vi "Status TCU Module.vi"(8 "error in (no error)":errorcluster, 11 "?":T1={"State"=enum."Idle", "Start Time"=timestamp(0 s since 1904-01-01), "Configuration"={"Cycle Period"=0.0, "Setpoint Entry"=0.0, "Output Device"=enum."Default", "Huber Ministat 230 Settings"={"VISA resource name"="", "Simulated?"=FALSE}, "Lauda Settings"={"VISA resource name"="", "Simulated?"=FALSE, "Pump Power"=2}, "Julabo FP-50 Settings"={"VISA resource name"="", "Simulated?"=FALSE, "Pump Power"=2}, "Internal Control?"=FALSE, "Huber Unistat 410 Settings"={"VISA resource name"="", "Address"=0, "Simulated?"=FALSE}}, "Current Time"=timestamp(0 s since 1904-01-01), "First Iteration"=FALSE, "Data"={"TCU Speed"=0.0, "Temperature"=0.0}, "Process Name"="", "TCU On?"=FALSE, "Output Error"=FALSE, "Start Log"=FALSE, "Power Level Changed"=FALSE} {"Configuration"."Huber Unistat 410 Settings"."Address" min=0 max=99 format="%02.0f"; "Configuration"."Julabo FP-50 Settings"."Pump Power" min=0 max=8 step=1; "Configuration"."Lauda Settings"."Pump Power" min=0 max=8 step=1}) -> (0 "error out":errorcluster, 3 "State out":T1={"State"=enum."Idle", "Start Time"=timestamp(0 s since 1904-01-01), "Configuration"={"Cycle Period"=0.0, "Setpoint Entry"=0.0, "Output Device"=enum."Huber Ministat 230", "Huber Ministat 230 Settings"={"VISA resource name"="", "Simulated?"=FALSE}, "Lauda Settings"={"VISA resource name"="", "Simulated?"=FALSE, "Pump Power"=2}, "Julabo FP-50 Settings"={"VISA resource name"="", "Simulated?"=FALSE, "Pump Power"=2}, "Internal Control?"=FALSE, "Huber Unistat 410 Settings"={"VISA resource name"="", "Address"=0, "Simulated?"=FALSE}}, "Current Time"=timestamp(0 s since 1904-01-01), "First Iteration"=FALSE, "Data"={"TCU Speed"=0.0, "Temperature"=0.0}, "Process Name"="", "TCU On?"=FALSE, "Output Error"=FALSE, "Start Log"=FALSE, "Power Level Changed"=FALSE} {"Configuration"."Huber Unistat 410 Settings"."Address" min=0 max=99 format="%02.0f"; "Configuration"."Julabo FP-50 Settings"."Pump Power" min=0 max=8 step=1; "Configuration"."Lauda Settings"."Pump Power" min=0 max=8 step=1})   [LabVIEW 2018, in "TCU Module.lvlib" / "TCU Module Engine.lvlib"]
uses:
  Measure Instrument/TCU Module Engine.lvlib
  Measure Instrument/TCU State Cluster.ctl
  Measure Instrument/State Enum.ctl
  TCU Module Settings Cluster.ctl
  Measure Instrument/Output Devices.ctl
  Huber TCU/Huber Settings.ctl
  Lauda Integral XT-150 TCU/Lauda Settings.ctl
  Julabo Type 1 TCU/Julabo Type 1 TCU Folder/Julabo FP-50 Settings.ctl
  Huber Unistat 410 TCU/Huber Unistat 410 RS485 Settings.ctl
  Tag VIs/Tag FGV Operation Enum.ctl
  Shared Variables/Dynamic Shared Variables.lvlib
  Huber TCU/Huber Ministat 230 TCU.lvlib
  Lauda Integral XT-150 TCU/Lauda TCU.lvlib
  Julabo Type 1 TCU/Julabo Type 1 TCU Folder/Julabo Type FP-50 TCU.lvlib
  Huber Unistat 410 TCU/Huber Unistat 410 TCU.lvlib
  TCU Module.lvlib
panel:
  # "Output Instruments"
  # "Output Instruments"
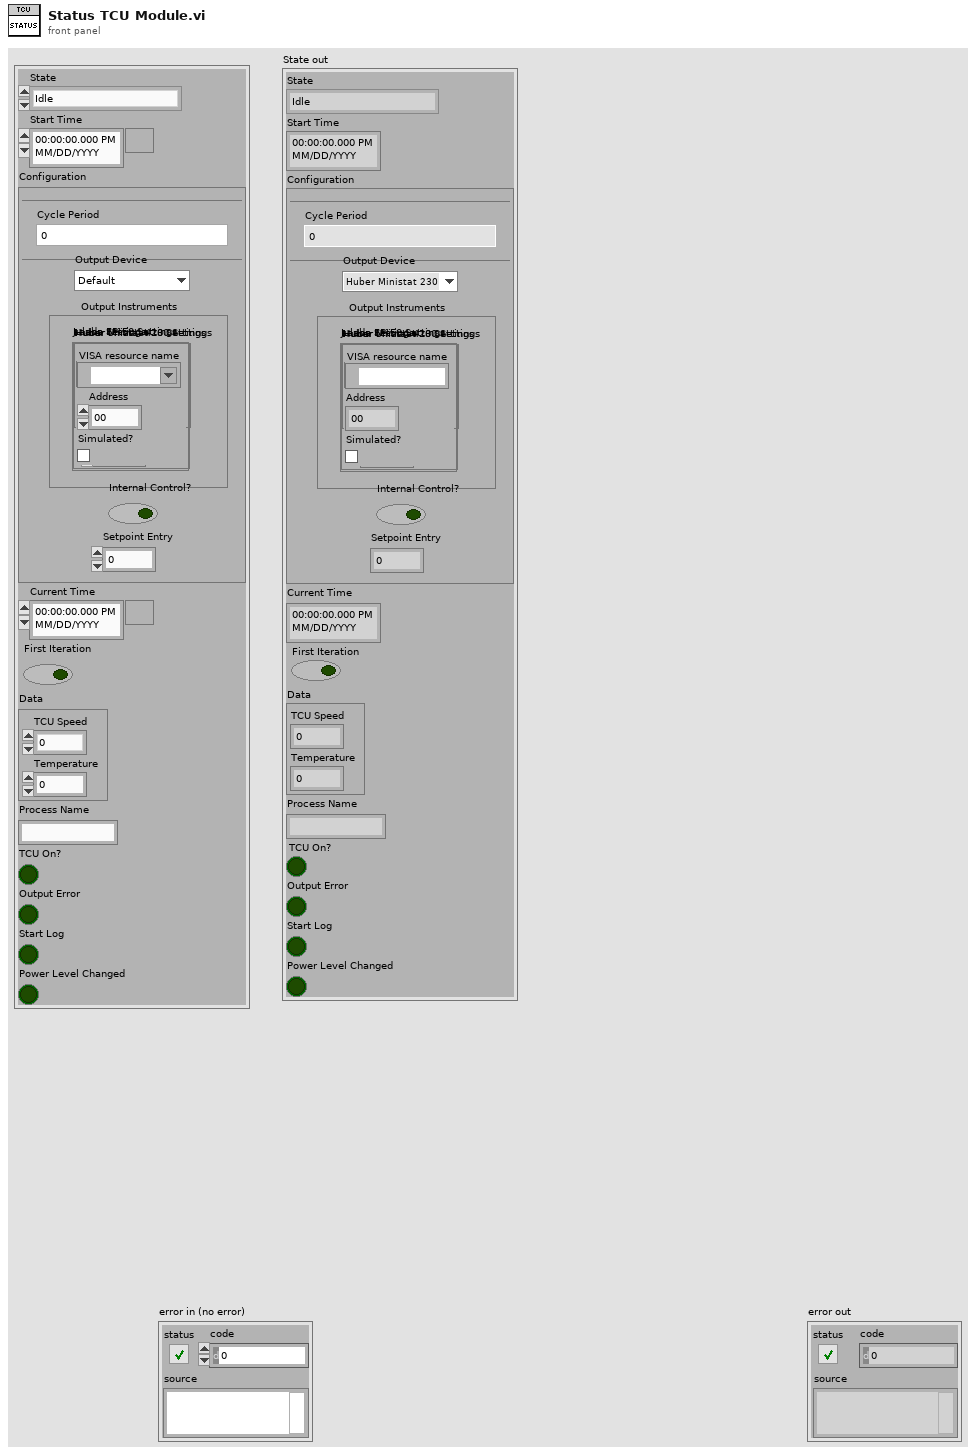
[diagram p1: front panel]
types:
  T1 = typedef "TCU Module.lvlib/TCU Module Engine.lvlib/TCU State Cluster.ctl" = cluster{"State":T2, "Start Time":timestamp, "Configuration":T3, "Current Time":timestamp, "First Iteration":bool, "Data":cluster{"TCU Speed":dbl, "Temperature":dbl}, "Process Name":string, "TCU On?":bool, "Output Error":bool, "Start Log":bool, "Power Level Changed":bool}
  T2 = typedef "TCU Module.lvlib/TCU Module Engine.lvlib/State Enum.ctl" = enum16{"Measuring", "Idle", "Paused"}
  T3 = typedef "TCU Module.lvlib/TCU Module Settings Cluster.ctl" = cluster{"Cycle Period":dbl, "Setpoint Entry":dbl, "Output Device":T4, "Huber Ministat 230 Settings":T5, "Lauda Settings":T6, "Julabo FP-50 Settings":T7, "Internal Control?":bool, "Huber Unistat 410 Settings":T8}
  T4 = typedef "Output Devices.ctl" = enum16{"Default", "Huber Ministat 230", "Huber Unistat 410", "Lauda XT-150", "Julabo FP-50"}
  T5 = typedef "Huber Ministat 230 TCU.lvlib/Huber Settings.ctl" = cluster{"VISA resource name":refnum<visa-resource-name>, "Simulated?":bool}
  T6 = typedef "Lauda TCU.lvlib/Lauda Settings.ctl" = cluster{"VISA resource name":refnum<visa-resource-name>, "Simulated?":bool, "Pump Power":i32}
  T7 = typedef "Julabo Type FP-50 TCU.lvlib/Julabo FP-50 Settings.ctl" = cluster{"VISA resource name":refnum<visa-resource-name>, "Simulated?":bool, "Pump Power":i32}
  T8 = typedef "Huber Unistat 410 TCU.lvlib/Huber Unistat 410 RS485 Settings.ctl" = cluster{"VISA resource name":refnum<visa-resource-name>, "Address":i8, "Simulated?":bool}
  T9 = typedef "Tag FGV Operation Enum.ctl" = enum16{"Init", "Set Notification Queue", "Create Tag", "Commit", "Write Tag (Numeric)", "Write Tag (Boolean)", "Read All Tags", "Read One Tag", "Delete Tag Category", "Set Alarm Parameters (Numeric)", "Set Alarm Parameters (Boolean)", "Enable All Alarms", "Disable All Alarms", "Delete All Tags", "Read Alarms", "Ack Alarm", "Read Alarm Parameters (Numeric)", "Read Alarm Parameters (Boolean)"}
  T10 = typedef "TCU Module.lvlib/TCU Module Tag Names Cluster.ctl" = cluster{"TCU Temp":string, "Output Device Tag":string, "TCU Speed":string, "Identifier Tag":string}
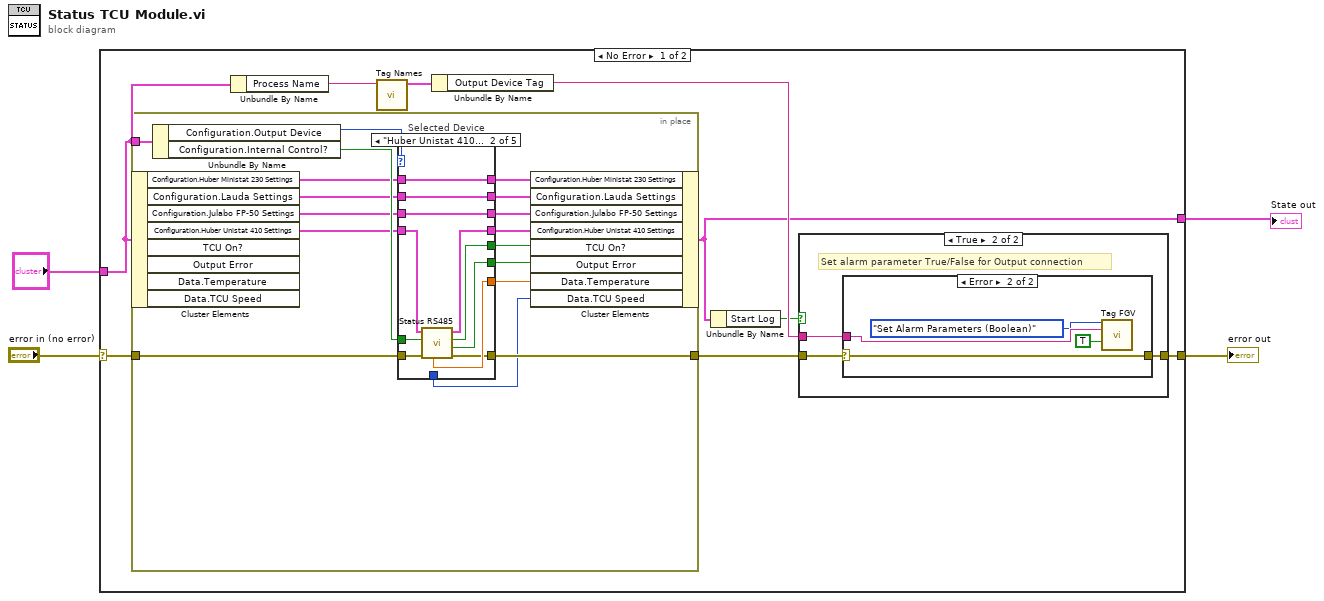
[diagram p0: block diagram]
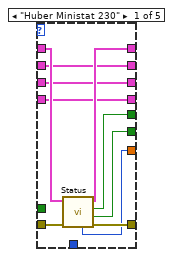
[diagram p2: hidden frame]
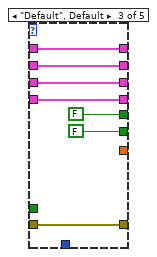
[diagram p3: hidden frame]
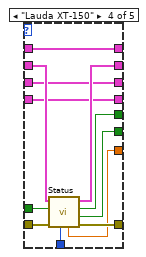
[diagram p4: hidden frame]
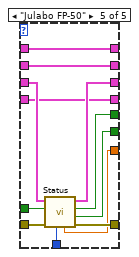
[diagram p5: hidden frame]
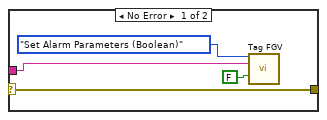
[diagram p7: hidden frame]
diagram:
  n1 = case shown="No Error" "error in (no error)" {
    selector: "error in (no error)" -> [w13 w96]
    tunnel: [w10 w96] -> w3
    tunnel: "?" -> [w6 w95]
    tunnel: [w5 w95] -> w1
    frame No Error {
      n2 = in-place {
        in-place-border: w13 -> [w30]
        in-place-border: [w29] -> w11
        in-place-border: w6 -> [w27]
        n3 = in-place-cluster #1(w6) -> ("Configuration.Huber Ministat 230 Settings"=w17:T5, "Configuration.Lauda Settings"=w16:T6, "Configuration.Julabo FP-50 Settings"=w15:T7, "Configuration.Huber Unistat 410 Settings"=w14:T8)  [unwired: 4 out]
        n4 = Unbundle By Name(w27) -> ("Configuration.Output Device"=w28:T4, "Configuration.Internal Control?"=w26:bool)
        n5 = case "Selected Device" shown="\"Huber Unistat 410\"" w28 {
          tunnel: w17 -> [w40 w51 w55 w63 w82]
          tunnel: [w38 w44 w58 w69 w79] -> w29
          tunnel: w30 -> [w39 w46 w58 w70 w80]
          tunnel: [w37 w42 FALSE w68 w76] -> w21
          tunnel: [w36 w41 FALSE ("Connection Error") w67 w75] -> w20
          tunnel: [w35 w51 w55 w63 w82] -> w25
          tunnel: [w34 w50 w54 w66 w81] -> w24
          tunnel: w16 -> [w34 w50 w54 w65 w81]
          tunnel: [w33 w49 w53 w64 w77] -> w23
          tunnel: w15 -> [w33 w49 w53 w64 w78]
          tunnel: [w31 w45 _ w62 w74] -> w19
          tunnel: [_ _ _ w61 w73] -> w18
          tunnel: w26 -> [_ w47 _ w60 w71]
          tunnel: [w32 w43 w52 w59 w72] -> w22
          tunnel: w14 -> [w32 w48 w52 w59 w72]
          frame "Huber Ministat 230" {
            n6 = call "Status.vi"("error in (no error)"=w39, "Huber Settings In"=w40) -> ("error out"=w38:errorcluster, "Connection Error"=w36:bool, "Running"=w37:bool, "Huber Settings Out"=w35:T5, "Temp"=w31:i32)  [unwired: 5 in]
          }
          frame "Huber Unistat 410" {
            n7 = call "Status RS485.vi"("error in (no error)"=w46, "Internal?"=w47, "Huber Unistat 410 Settings"=w48) -> ("error out"=w44:errorcluster, "Connection Error"=w41:bool, "Running"=w42:bool, "Huber Unistat 410 Settings"=w43:T8, "Temperature"=w45:dbl)  [unwired: 4 in]
          }
          frame "Default", Default {
          }
          frame "Lauda XT-150" {
            n8 = call "Status.vi"("error in (no error)"=w70, "Internal?"=w60, "Lauda Settings"=w65) -> ("error out"=w69:errorcluster, "Connection Error"=w67:bool, "Running"=w68:bool, "Lauda Settings"=w66:T6, "Temp"=w62:dbl, "Pump Speed"=w61:i32)  [unwired: 2 in, 1 out]
          }
          frame "Julabo FP-50" {
            n9 = call "Status.vi"("error in (no error)"=w80, "Internal?"=w71, "Julabo FP-50 Settings In"=w78) -> ("error out"=w79:errorcluster, "Connection Error"=w75:bool, "Running"=w76:bool, "Julabo FP-50 Settings Out"=w77:T7, "Temp"=w74:dbl, "Pumpstage (out)"=w73:u8)  [unwired: 3 in]
          }
        }
        n10 = in-place-cluster #1("Configuration.Huber Ministat 230 Settings"=w25, "Configuration.Lauda Settings"=w24, "Configuration.Julabo FP-50 Settings"=w23, "Configuration.Huber Unistat 410 Settings"=w22, "TCU On?"=w21, "Output Error"=w20, "Data.Temperature"=w19, "Data.TCU Speed"=w18) -> (w5:T1)
      }
      n11 = Unbundle By Name(w6) -> ("Process Name"=w8:string)
      n12 = call "Tag Names.vi"("Process Name"=w8) -> ("Pump Module Tag Names"=w9:T10)  [unwired: 8 in, 2 out]
      n13 = Unbundle By Name(w9) -> ("Output Device Tag"=w12:string)
      n14 = Unbundle By Name(w5) -> ("Start Log"=w7:bool)
      n15 = case shown="True" w7 {
        tunnel: w12 -> [_ w86]
        tunnel: w11 -> [w83 w85]
        tunnel: [w83 w84] -> w10
        frame False {
        }
        frame True {
          # "Set alarm parameter True/False for Output connection"
          n16 = case shown="Error" w85 {
            selector: w85 -> [w90 w94]
            tunnel: [w90 w94] -> w84
            tunnel: w86 -> [w87 w93]
            frame No Error {
              n17 = call "Tag FGV.vi"("Operation"=Tag_FGV_Operation_Enum."Set Alarm Parameters (Boolean)", "Tag Name"=w87, "Data"=FALSE) -> ()  [unwired: 5 in, 8 out]
            }
            frame Error {
              n18 = call "Tag FGV.vi"("Operation"=Tag_FGV_Operation_Enum."Set Alarm Parameters (Boolean)", "Tag Name"=w93, "Data"=TRUE) -> ()  [unwired: 5 in, 8 out]
            }
          }
        }
      }
    }
    frame Error {
    }
  }
  "error out" <- w3
  "State out" <- w1
